vi "ButtonHold6Totes.vi"(11 "Buttons":bool[](array[boolean])) -> ()   [LabVIEW 2014]
uses:
  Gantry/GantryGlobals.vi
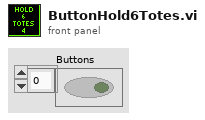
[diagram p1: front panel]
types:
  T1 = enum16{"WaitForInput", "LowerLift", "OpenArms", "RaiseLift", "CloseArms"}
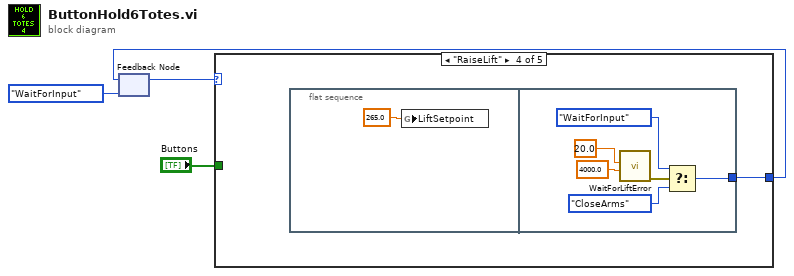
[diagram p0: block diagram]
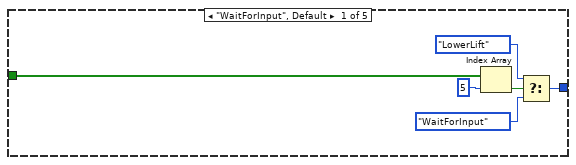
[diagram p2: hidden frame]
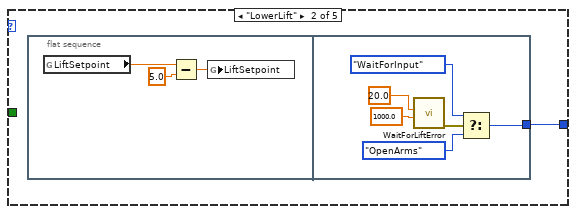
[diagram p3: hidden frame]
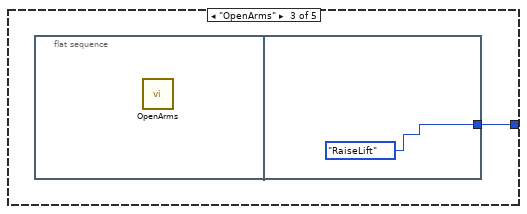
[diagram p4: hidden frame]
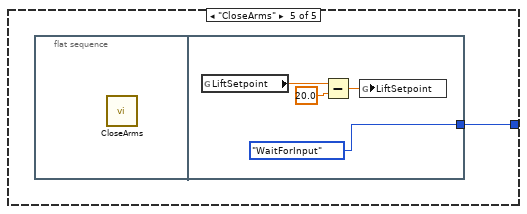
[diagram p5: hidden frame]
diagram:
  n1 = feedback #1(T1."WaitForInput" ("Enum")) -> (w1:T1)
  n2 = case shown="\"RaiseLift\"" w1 {
    tunnel: [w9 w11 w21 w23 w31] -> w3
    tunnel: "Buttons" -> [w7 _ _ _ _]
    frame "WaitForInput", Default {
      n3 = Index Array(array=w7, index=5) -> (element=w5:bool)
      n4 = Select(t=T1."LowerLift" ("Enum"), s=w5, f=T1."WaitForInput" ("Enum")) -> (s? t:f=w9:T1)
    }
    frame "LowerLift" {
      n5 = flat-sequence {
        tunnel: [w15] -> w11
        frame #0 {
          n6 = global read "GantryGlobals.vi" "LiftSetpoint"() -> (w14:dbl)
          n7 = Subtract(x=w14, y=5.0) -> (x-y=w13:dbl)
          n8 = global write "GantryGlobals.vi" "LiftSetpoint"(w13) -> ()
        }
        frame #1 {
          n9 = call "WaitForLiftError.vi"("Timeout (ms)"=1000.0, "AllowedError"=20.0) -> ("error out"=w20:errorcluster)  [unwired: 9 in]
          n10 = Select(t=T1."WaitForInput" ("Enum"), s=w20, f=T1."OpenArms" ("Enum")) -> (s? t:f=w15:T1)
        }
      }
    }
    frame "OpenArms" {
      n11 = flat-sequence {
        tunnel: [T1."RaiseLift" ("Enum")] -> w21
        frame #0 {
          n12 = call "OpenArms.vi"() -> ()  [unwired: 12 in]
        }
        frame #1 {
        }
      }
    }
    frame "RaiseLift" {
      n13 = flat-sequence {
        tunnel: [w25] -> w23
        frame #0 {
          n14 = global write "GantryGlobals.vi" "LiftSetpoint"(265.0 ("LiftSetpoint")) -> ()
        }
        frame #1 {
          n15 = call "WaitForLiftError.vi"("Timeout (ms)"=4000.0, "AllowedError"=20.0) -> ("error out"=w30:errorcluster)  [unwired: 9 in]
          n16 = Select(t=T1."WaitForInput" ("Enum"), s=w30, f=T1."CloseArms" ("Enum")) -> (s? t:f=w25:T1)
        }
      }
    }
    frame "CloseArms" {
      n17 = flat-sequence {
        tunnel: [T1."WaitForInput" ("Enum")] -> w31
        frame #0 {
          n18 = call "CloseArms.vi"() -> ()  [unwired: 12 in]
        }
        frame #1 {
          n19 = global read "GantryGlobals.vi" "LiftSetpoint"() -> (w34:dbl)
          n20 = Subtract(x=w34, y=20.0) -> (x-y=w33:dbl)
          n21 = global write "GantryGlobals.vi" "LiftSetpoint"(w33) -> ()
        }
      }
    }
  }
  n22 = feedback-in #1(w3) -> ()
